vi "write pair information.vi"(8 "error in":errorcluster, 10 "pair info":T1, 11 "UDP Broadcast Editor Node in":refnum<class "TEC editor node.lvclass">) -> (0 "error out":errorcluster, 3 "UDP Broadcast Editor Node out":refnum<class "TEC editor node.lvclass">)   [LabVIEW 2014, in "TEC editor node.lvclass"]
uses:
  TEC editor node.lvclass
  pair information.ctl
  TEC editor node.lvclass/TEC editor node.ctl
  <vilib>/NI/Configuration Framework/serializable configuration/NISE_CEF_serializable configuration.lvclass
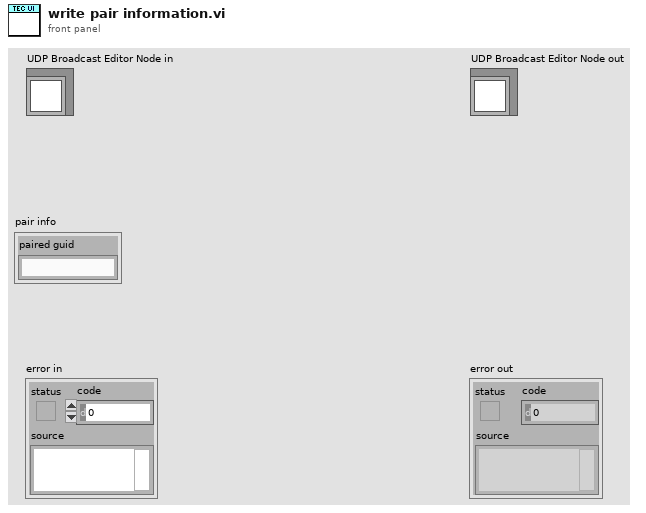
[diagram p1: front panel]
types:
  T1 = typedef "TEC editor node.lvclass/pair information.ctl" = cluster{"paired guid":string}
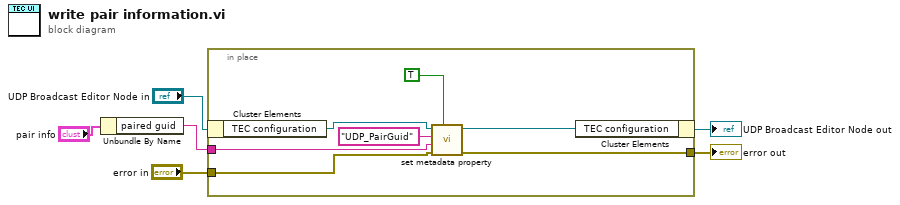
[diagram p0: block diagram]
diagram:
  n1 = Unbundle By Name("pair info") -> ("paired guid"=w1:string)
  n2 = in-place {
    in-place-border: "error in" -> [w11]
    in-place-border: [w7] -> w3
    in-place-border: w1 -> [w8]
    n3 = in-place-cluster #1("UDP Broadcast Editor Node in") -> ("TEC configuration"=w13:refnum<class "TEC configuration.lvclass">)
    n4 = call <vilib>:"set metadata property.vi"("overwrite?"=TRUE, "error in"=w11, "value"=w8, "key"="UDP_PairGuid", "configuration in"=w13) -> ("error out"=w7:errorcluster, "configuration out"=w12:refnum<class "TEC configuration.lvclass">)  [unwired: 5 in]
    n5 = in-place-cluster #1("TEC configuration"=w12) -> (→"UDP Broadcast Editor Node out":refnum<class "TEC editor node.lvclass">)
  }
  "error out" <- w3
